vi "Pre Launch Init.vi"(11 "ParentActor in":refnum<class "ParentActor.lvclass"> caption="操作者输入") -> (0 "error out":errorcluster caption="错误输出", 3 "ParentActor out":refnum<class "ParentActor.lvclass"> caption="操作者输出")   [LabVIEW 2014, in "UnitTest.lvlib" / "ParentActor.lvclass"]
doc: "(<B>Filename</B>: Actor Framework.lvlib:Actor.lvclass:Pre Launch Init.vi)\n\nDefines behavior that occurs after the Launch Nested Actor method is invoked but before the actor's Actor Core method begins running.\n\nBy default, this method does nothing. A descendant class may override it to define behavior."
uses:
  ParentActor.lvclass
  labview/1603/zsRobotSynergeticSystem/zsLib/zsActor/zsActor.lvclass
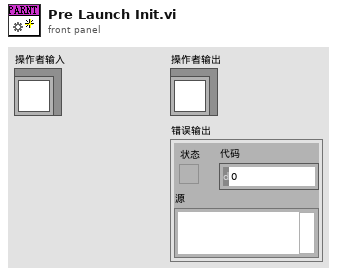
[diagram p1: front panel]
types:
  T1 = enum16{"OpenSlaveActor", "Idle", "StopSlaveActor"}
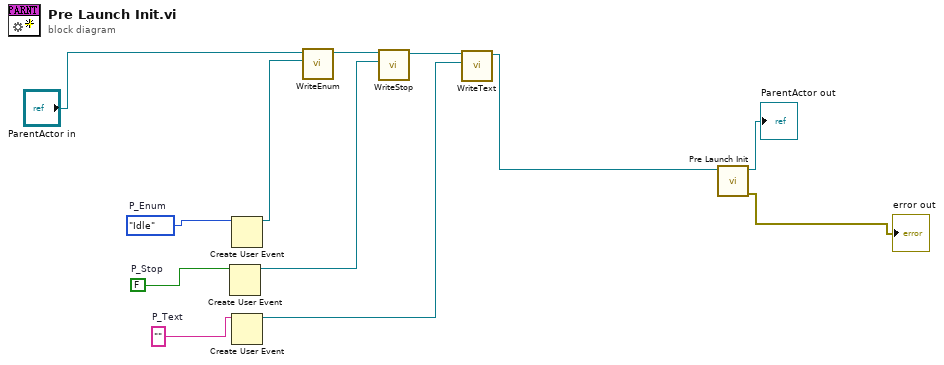
[diagram p0: block diagram]
diagram:
  w9 = ""  # P_Text
  w10 = FALSE  # P_Stop
  w11 = T1."Idle"  # P_Enum
  n1 = Create User Event(user event datatype=w10) -> (user event=w4:refnum<user-event>)  [unwired: 1 in, 1 out]
  n2 = Create User Event(user event datatype=w11) -> (user event=w7:refnum<user-event>)  [unwired: 1 in, 1 out]
  n3 = Create User Event(user event datatype=w9) -> (user event=w3:refnum<user-event>)  [unwired: 1 in, 1 out]
  n4 = call-dynamic "WriteEnum.vi"("Enum"=w7, "zsActor输入"="ParentActor in") -> ("zsActor输出"=w6:refnum<class "ParentActor.lvclass">)  [unwired: 8 in, 1 out]
  n5 = call-dynamic "WriteStop.vi"("Stop"=w4, "zsActor输入"=w6) -> ("zsActor输出"=w5:refnum<class "ParentActor.lvclass">)  [unwired: 8 in, 1 out]
  n6 = call-dynamic "WriteText.vi"("Text"=w3, "zsActor输入"=w5) -> ("zsActor输出"=w2:refnum<class "ParentActor.lvclass">)  [unwired: 8 in, 1 out]
  n7 = call-parent "Pre Launch Init.vi"("Actor in"=w2) -> ("error out"=→"error out":errorcluster, "Actor out"=→"ParentActor out":refnum<class "ParentActor.lvclass">)  [unwired: 9 in]
